vi "ReadWrite.Data.Write.vi"(7 "Force":bool, 8 "error in":errorcluster, 9 "Offset":i32, 10 "Values":dbl[](array[numeric]), 11 "Ref":T1) -> (0 "error out":errorcluster)   [LabVIEW 2027, in "Data Access Engine.lvlib" / "Data Access Engine.lvclass"]
uses:
  Data Access Engine.lvclass
  Types/ReadWrite.DVR.ctl
  Access Type Classes/ReadWrite/ReadWrite.lvclass
  Access Type Classes/ReadWrite/ReadWrite.lvclass/ReadWrite.ctl
  Access Type Classes/ReadWrite/ReadWrite.ProcessData.Buffer.vi
  Access Type Classes/ReadWrite/ReadWrite.ProcessData.Commit.vi
  <vilib>/NI VeriStand/Custom Device API/NI VeriStand - Get Channel Value by Data Reference.vi
  <vilib>/NI VeriStand/Custom Device API/NI VeriStand - Set Channel Value by Data Reference.vi
  <vilib>/NI VeriStand/Custom Device API/Global Data Refs.vi
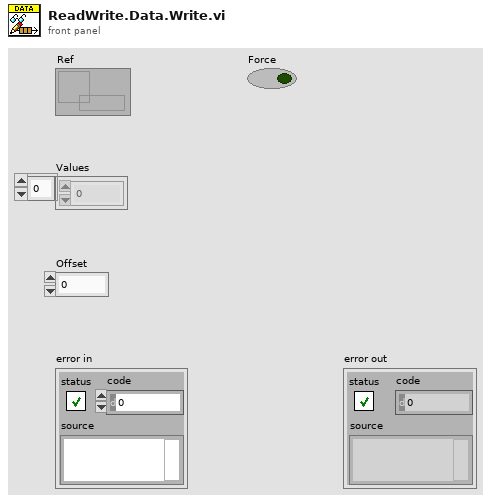
[diagram p1: front panel]
types:
  T1 = typedef "Data Access Engine.lvlib/Data Access Engine.lvclass/ReadWrite.DVR.ctl" = refnum<data-value>
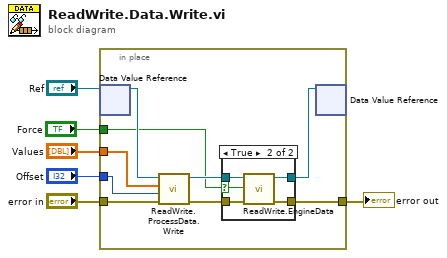
[diagram p0: block diagram]
diagram:
  n1 = in-place {
    in-place-border: "error in" -> [w15]
    in-place-border: [w13] -> w5
    in-place-border: "Values" -> [w11]
    in-place-border: "Offset" -> [w10]
    in-place-border: "Force" -> [w7]
    n2 = in-place-dvr #1("Ref") -> (w12:refnum<class "ReadWrite.lvclass">)  [unwired: 1 out]
    n3 = call "ReadWrite.ProcessData.Write.vi"("error in (no error)"=w15, "Offset"=w10, "Values"=w11, "ReadWrite in"=w12) -> ("error out"=w14:errorcluster, "ReadWrite out"=w9:refnum<class "ReadWrite.lvclass">)  [unwired: 5 in]
    n4 = case shown="True" w7 {
      selector: w7 -> [_ w18]
      tunnel: w14 -> [w17 w22]
      tunnel: [w17 w21] -> w13
      tunnel: w9 -> [w16 w20]
      tunnel: [w16 w19] -> w8
      frame False {
      }
      frame True {
        n5 = call "ReadWrite.EngineData.vi"("error in"=w22, "Force"=w18, "ReadWrite in"=w20) -> ("error out"=w21:errorcluster, "ReadWrite out"=w19:refnum<class "ReadWrite.lvclass">)  [unwired: 7 in]
      }
    }
    n6 = in-place-dvr #1(w8) -> ()  [unwired: 2 out]
  }
  "error out" <- w5
